vi "HV_mesura_Ileak.vi"(2 "VISA resource name":refnum<visa-resource-name>="GPIB1::25::INSTR", 3 "notifier Ileak":refnum<notifier>) -> ()   [LabVIEW 2015, in "VIPM2.lvlib"]
doc: "Executa segons notificacions les mesures de Ileak.\nEn acabar, grava CSV i les gràfiques en PNG dins de EQ folder path."
uses:
  VIPM2.lvlib
  dr_Keithley 24XX/Keithley 24XX.lvlib
panel:
  out "time":sgl
  out "barra":u8(slide) scale=0.0..5.0
  out "Waveform Graph":sgl[](graph)
  out "Chart":cluster{sgl, sgl}[](graph)
  out "Current":sgl format="%#_6p"
  out "Voltage":sgl
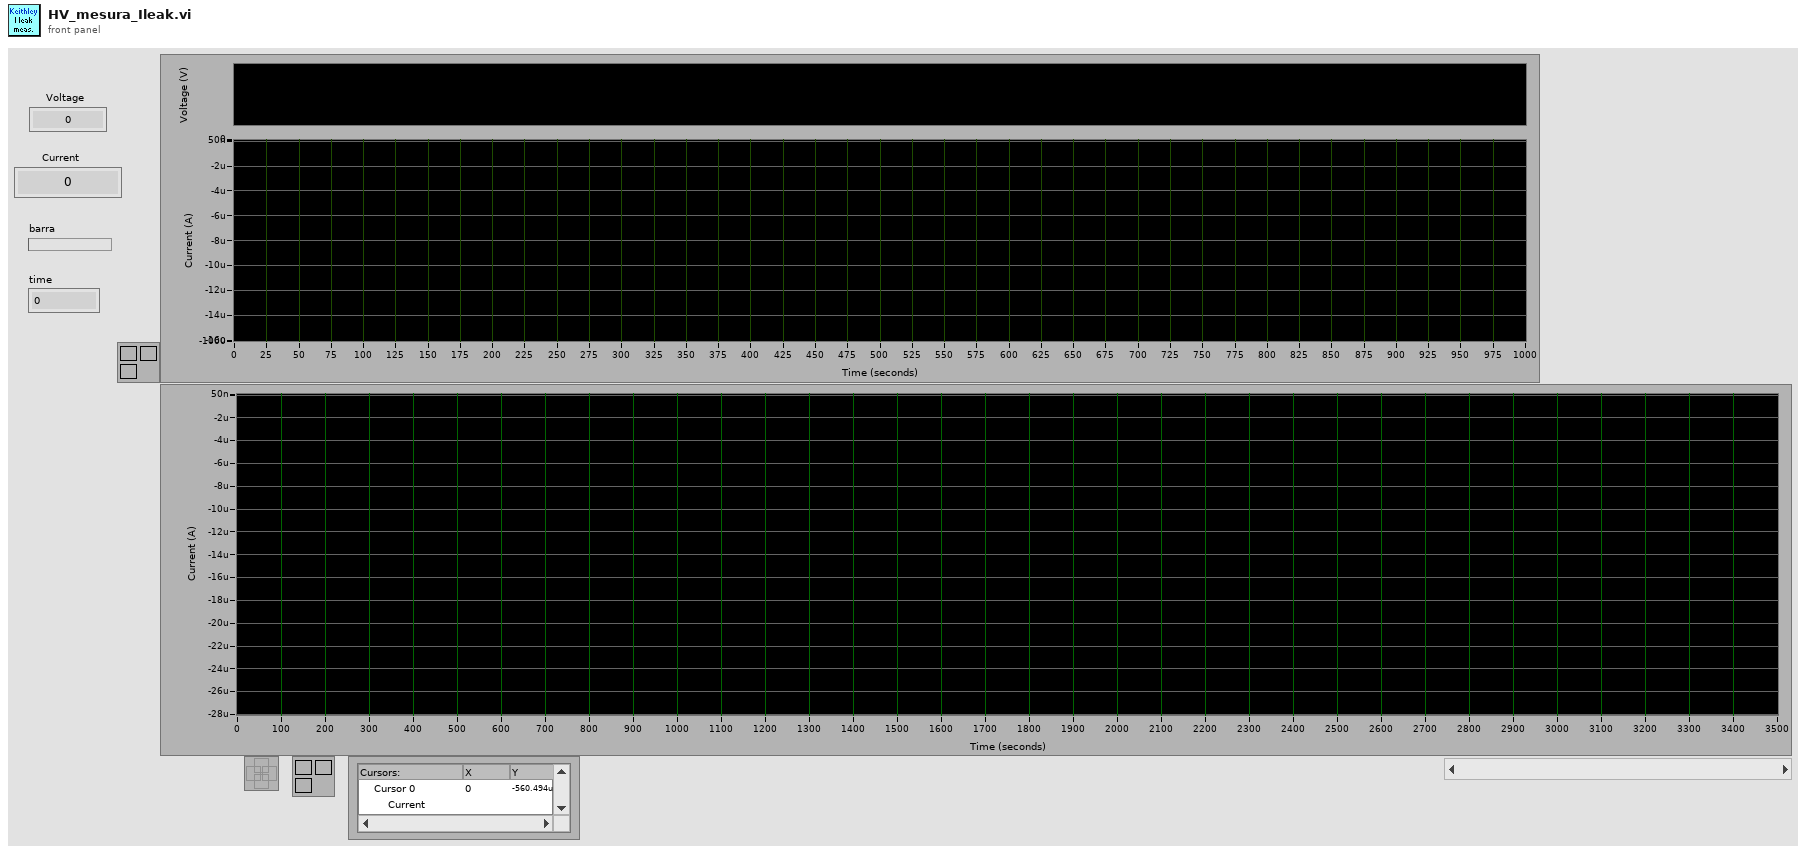
[diagram p1: front panel]
types:
  T1 = typedef "imagedata.ctl" = cluster{"image type":i32, "image depth":i32, "image":u8[], "mask":u8[], "colors":u32[], "Rectangle":cluster{"left":i16, "top":i16, "right":i16, "bottom":i16}}
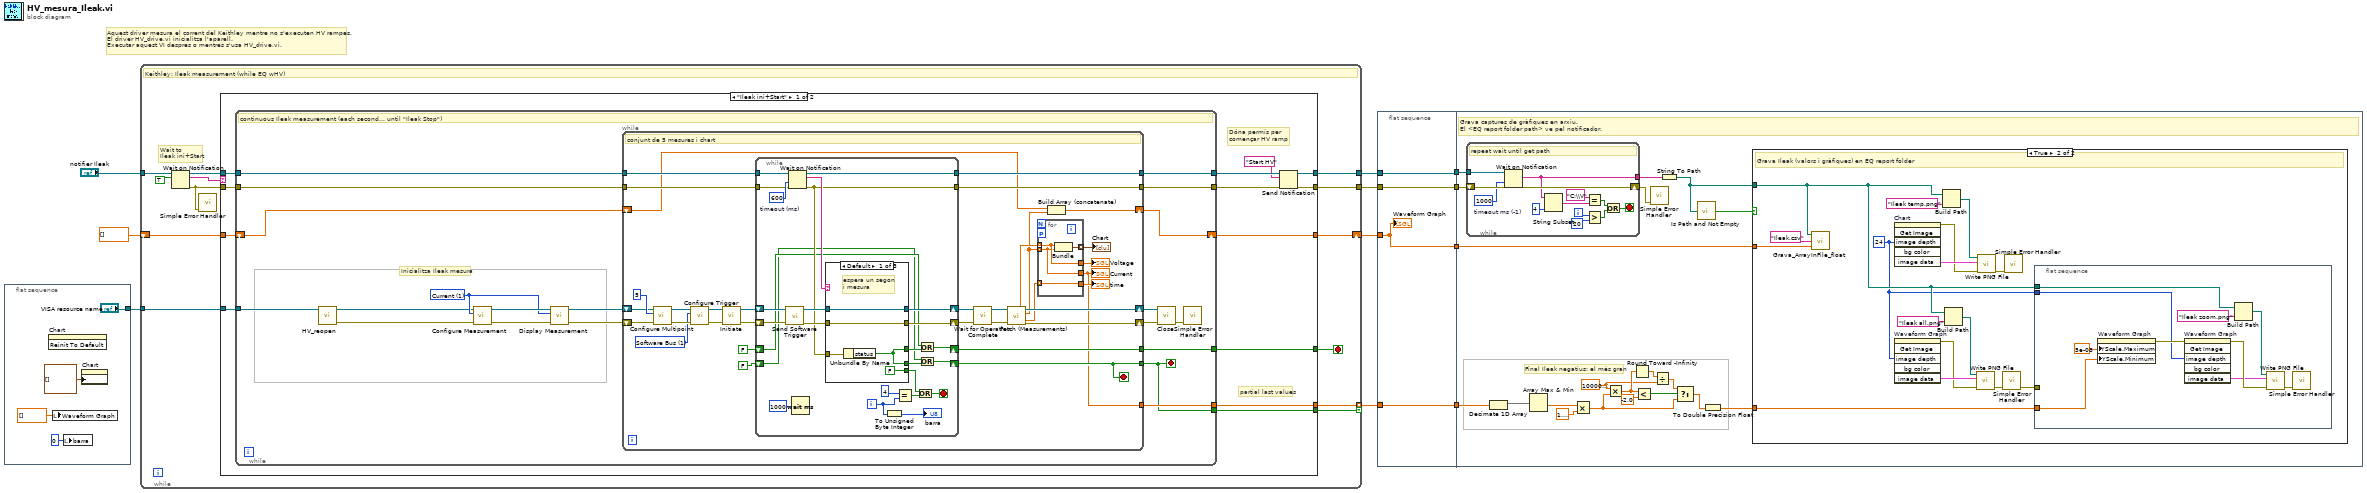
[diagram p0: block diagram]
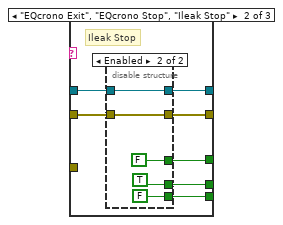
[diagram p3: hidden frame]
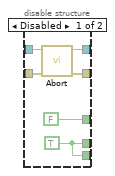
[diagram p4: hidden frame]
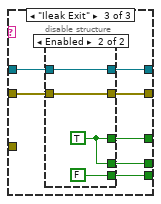
[diagram p5: hidden frame]
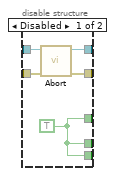
[diagram p6: hidden frame]
diagram:
  # "Aquest driver mesura el corrent del Keithley mentre no s'executen HV rampes.\nEl driver HV_drive.vi inicialitza l'aparell.\nExecutar aquest VI despres o mentres s'usa HV_drive.vi."
  n1 = flat-sequence {
    tunnel: ["VISA resource name"] -> w11
    frame #0 {
      n2 = invoke on="Chart" class="WFChart (strict)" method="Reinit To Default"() -> ()  [unwired: 3 in, 3 out]
      n3 = local write "Waveform Graph"(sgl[] [] ("Waveform Graph")) -> ()
      n4 = local write "barra"(u8 0 ("barra")) -> ()
      n5 = property on="Chart" class="WFChart (strict)"("History Data"=cluster{sgl, sgl}[] []) -> ()  [unwired: 2 in, 2 out]
    }
  }
  n6 = while {
    tunnel: w11 -> [w28]
    shift-right: [w27] -> w8
    shift-left: sgl[] [] -> [w26]
    tunnel: "notifier Ileak" -> [w25]
    tunnel: [w20] -> w7
    tunnel: [w19] -> w6
    tunnel: [w17] -> w2 mode=indexing if=w16
    stop <- w21 stop-if-true
    # "Wait to\nIleak ini+Start"
    # "Keithley: Ileak measurement (while EQ wHV)"
    n7 = Wait on Notification(notifier=w25, ignore previous (F)=TRUE) -> (notifier out=w22:refnum<notifier>, notification=w23:string, error out=w18:errorcluster)  [unwired: 2 in, 1 out]
    n8 = call <vilib>:"Simple Error Handler.vi"("error in (no error)"=w18) -> ()  [unwired: 4 in, 5 out]
    n9 = case shown="\"Ileak ini+Start\"" w23 {
      tunnel: w28 -> [w36 _]
      tunnel: [w41 w165] -> w27
      tunnel: w26 -> [w40 w165]
      tunnel: w22 -> [w39 w164]
      tunnel: w18 -> [w38 w163]
      tunnel: [w37 _] -> w21
      tunnel: [w34 w164] -> w20
      tunnel: [w32 w163] -> w19
      tunnel: [w30 _] -> w17
      tunnel: [w29 _] -> w16
      frame "Ileak ini+Start" {
        # "partial last values"
        # "Dóna permís per\ncomençar HV ramp"
        n10 = while {
          shift-right: [w57] -> w41
          shift-left: w40 -> [w55]
          tunnel: w39 -> [w61]
          tunnel: w38 -> [w60]
          tunnel: [w56] -> w37
          tunnel: [w59] -> w35
          tunnel: [w58] -> w33
          tunnel: w36 -> [w44]
          tunnel: [w46] -> w30
          tunnel: [w45] -> w29
          stop <- w45 stop-if-true
          w52 = u16 1 items=["Volts", "Current", "Resistance"] ("Function (0: Volts)")
          # "Inicialitza Ileak mesura"
          # "continuous Ileak measurement (each second... until \"Ileak Stop\")"
          n11 = call "HV_reopen.vi"("VISA resource name"=w44) -> ("error out"=w42:errorcluster, "VISA resource name out"=w43:refnum<visa-resource-name>)  [unwired: 9 in]
          n12 = call "Configure Measurement.vi"("error in (no error)"=w42, "Function (0: Volts)"=w52, "VISA resource name"=w43) -> ("error out"=w53:errorcluster, "VISA resource name out"=w54:refnum<visa-resource-name>)  [unwired: 7 in]
          n13 = call "Display Measurement.vi"("error in (no error)"=w53, "Displayed Measurement (0: Voltage)"=w52, "VISA resource name"=w54) -> ("error out"=w50:errorcluster, "VISA resource name out"=w51:refnum<visa-resource-name>)  [unwired: 7 in]
          n14 = while {
            tunnel: w61 -> [w76]
            tunnel: w60 -> [w75]
            tunnel: [w74] -> w59
            tunnel: [w73] -> w58
            tunnel: [w72] -> w56
            tunnel: [w71] -> w45
            shift-right: [w77] -> w57
            shift-left: w55 -> [w68]
            shift-right: [w94] -> w48
            shift-left: w51 -> [w67]
            shift-right: [w65] -> w47
            shift-left: w50 -> [w66]
            tunnel: [w64] -> w46
            stop <- w71 stop-if-true
            w91 = u16 1 items=["Immediate", "Software Bus", "Timer", "Manual", "Trigger Link", "Rising SOT Pulse", "Falling SOT Pulse", "Rising or Falling SOT Pulse"] ("Arming Source  (0: Immediate)")
            # "conjunt de 5 mesures i chart"
            n15 = call "Configure Multipoint.vi"("error in (no error)"=w66, "Number of Times to Arm (1)"=5 ("Trigger Count (1)"), "VISA resource name"=w67) -> ("error out"=w92:errorcluster, "VISA resource name out"=w93:refnum<visa-resource-name>)  [unwired: 7 in]
            n16 = call "Configure Trigger.vi"("error in (no error)"=w92, "Arming Source  (0: Immediate)"=w91, "VISA resource name"=w93) -> ("error out"=w89:errorcluster, "VISA resource name out"=w90:refnum<visa-resource-name>)  [unwired: 7 in]
            n17 = call "Initiate.vi"("error in (no error)"=w89, "VISA resource name"=w90) -> ("error out"=w87:errorcluster, "VISA resource name out"=w88:refnum<visa-resource-name>)  [unwired: 8 in]
            n18 = while {
              shift-right: [w104] -> w86
              shift-left: w88 -> [w118]
              shift-right: [w103] -> w85
              shift-left: w87 -> [w117]
              tunnel: w76 -> [w110]
              tunnel: w75 -> [w109]
              tunnel: [w107] -> w74
              tunnel: [w102] -> w73
              shift-right: [w98] -> w72
              shift-left: FALSE -> [w99]
              shift-right: [w95] -> w71
              shift-left: FALSE -> [w96]
              i -> [w113]
              stop <- w115 stop-if-true
              w111 = 600  # timeout (ms)
              n19 = call "Send Software Trigger.vi"("error in (no error)"=w117, "VISA resource name"=w118) -> ("error out"=w105:errorcluster, "VISA resource name out"=w106:refnum<visa-resource-name>)  [unwired: 8 in]
              n20 = Wait on Notification(notifier=w110, timeout in ms (-1)=w111, error in (no error)=w109) -> (notifier out=w107:refnum<notifier>, notification=w108:string, error out=w102:errorcluster)  [unwired: 1 in, 1 out]
              n21 = Wait (ms)(milliseconds to wait=u32 1000 ("millisecond multiple")) -> ()  [unwired: 1 out]
              n22 = case shown="Default" w108 {
                tunnel: w102 -> [w124 _ _]
                tunnel: [w121 w127 w145] -> w100
                tunnel: [w121 w126 w144] -> w97
                tunnel: w106 -> [w123 w131 w149]
                tunnel: w105 -> [w122 w130 w147]
                tunnel: [w123 w129 w148] -> w104
                tunnel: [w122 w128 w146] -> w103
                tunnel: [FALSE w125 w143] -> w101
                frame Default {
                  # "espera un segon\ni mesura"
                  n23 = Unbundle By Name(w124) -> ("status"=w121:bool)
                }
                frame "EQcrono Exit", "EQcrono Stop", "Ileak Stop" {
                  # "Ileak Stop"
                  n24 = disable-structure shown="Enabled" {
                    disable-tunnel: w131 -> [w137 w142]
                    disable-tunnel: w130 -> [w136 w141]
                    disable-tunnel: [w135 w142] -> w129
                    disable-tunnel: [w134 w141] -> w128
                    disable-tunnel: [FALSE FALSE] -> w127
                    disable-tunnel: [w132 TRUE] -> w126
                    disable-tunnel: [w132 FALSE] -> w125
                    frame Disabled {
                      w132 = TRUE
                      n25 = call "Abort.vi"("error in (no error)"=w136, "VISA resource name"=w137) -> ("error out"=w134:errorcluster, "VISA resource name out"=w135:refnum<visa-resource-name>)  [unwired: 8 in]
                    }
                    frame Enabled {
                    }
                  }
                }
                frame "Ileak Exit" {
                  n26 = disable-structure shown="Enabled" {
                    disable-tunnel: w149 -> [w154 w158]
                    disable-tunnel: [w153 w158] -> w148
                    disable-tunnel: w147 -> [w152 w157]
                    disable-tunnel: [w151 w157] -> w146
                    disable-tunnel: [w150 w156] -> w145
                    disable-tunnel: [w150 w156] -> w144
                    disable-tunnel: [w150 FALSE] -> w143
                    frame Disabled {
                      w150 = TRUE
                      n27 = call "Abort.vi"("error in (no error)"=w152, "VISA resource name"=w154) -> ("error out"=w151:errorcluster, "VISA resource name out"=w153:refnum<visa-resource-name>)  [unwired: 8 in]
                    }
                    frame Enabled {
                      w156 = TRUE
                    }
                  }
                }
              }
              n28 = To Unsigned Byte Integer(number=w113) -> (unsigned 8bit integer=→"barra":u8)
              n29 = Equal?(x=4 ("y"), y=w113) -> (x = y?=w116:bool)
              n30 = Or(x=w101, y=w116) -> (x .or. y?=w115:bool)
              n31 = Or(x=w96, y=w97) -> (x .or. y?=w95:bool)
              n32 = Or(x=w99, y=w100) -> (x .or. y?=w98:bool)
            }
            n33 = call "Wait for Operation Complete.vi"("error in (no error)"=w85, "VISA resource name"=w86) -> ("error out"=w83:errorcluster, "VISA resource name out"=w84:refnum<visa-resource-name>)  [unwired: 8 in]
            n34 = call "Fetch (Measurements).vi"("VISA resource name"=w84, "error in (no error)"=w83) -> ("Voltage"=w81:sgl[], "VISA resource name out"=w94:refnum<visa-resource-name>, "Current"=w78:sgl[], "Timestamp"=w70:sgl[], "error out"=w65:errorcluster)  [unwired: 7 in, 2 out]
            n35 = for {
              tunnel: w81 -> [w161] mode=indexing
              tunnel: w78 -> [w160] mode=indexing
              tunnel: [w162] -> w80 mode=indexing
              tunnel: [w161] -> w79
              tunnel: [w160] -> w64
              tunnel: w70 -> [w159] mode=indexing
              tunnel: [w159] -> w69
              workers-P: _ -> [_]
              n36 = Bundle(w161, w160) -> (w162:cluster{sgl, sgl})  [unwired: 1 in]
            }
            "Chart" <- w80
            "Voltage" <- w79
            "Current" <- w64
            "time" <- w69
            n37 = Build Array (concatenate) "Build Array"(w68, w78) -> (w77:sgl[])
          }
          n38 = call "Close.vi"("error in (no error)"=w47, "VISA resource name"=w48) -> ("error out"=w49:errorcluster)  [unwired: 9 in]
          n39 = call <vilib>:"Simple Error Handler.vi"("error in (no error)"=w49) -> ()  [unwired: 4 in, 5 out]
        }
        n40 = Send Notification(notification="Start HV", notifier=w35, error in (no error)=w33) -> (notifier out=w34:refnum<notifier>, error out=w32:errorcluster)
      }
      frame Default {
      }
    }
  }
  n41 = flat-sequence {
    tunnel: w8 -> [w167]
    tunnel: w7 -> [w169]
    tunnel: w6 -> [w168]
    tunnel: [w169] -> w5
    tunnel: [w168] -> w4
    tunnel: [w167] -> w3
    tunnel: w2 -> [w166]
    tunnel: [w166] -> w1
    tunnel: w5 -> [w189]
    tunnel: w4 -> [w188]
    tunnel: w3 -> [w184]
    tunnel: w1 -> [w182]
    frame #0 {
      "Waveform Graph" <- w167
    }
    frame #1 {
      w173 = sgl 1000000.0 ("x")
      # "Final Ileak negatius: el més gran"
      # "Grava captures de gràfiques en arxiu.\nEl <EQ report folder path> ve pel notificador."
      n42 = while {
        tunnel: w189 -> [w202]
        tunnel: [w198] -> w186
        shift-right: [w199] -> w187
        shift-left: w188 -> [w201]
        i -> [w194]
        stop <- w190 stop-if-true
        w200 = 1000  # timeout ms (-1)
        # "repeat wait until get path"
        n43 = Wait on Notification(notifier=w202, timeout in ms (-1)=w200, error in (no error)=w201) -> (notification=w198:string, error out=w199:errorcluster)  [unwired: 1 in, 2 out]
        n44 = String Subset(string=w198, length (rest)=4 ("length (rest)")) -> (substring=w196:string)  [unwired: 1 in]
        n45 = Equal?(x="C:\\V", y=w196) -> (x = y?=w191:bool)
        n46 = Greater?(x=w194, y=20) -> (0:w192:bool)
        n47 = Or(x=w191, y=w192) -> (x .or. y?=w190:bool)
      }
      n48 = Decimate 1D Array "Decimate 1D Array"(w182) -> (w181:sgl[])  [unwired: 1 out]
      n49 = Array Max & Min(array=w181) -> (min value=w180:sgl)  [unwired: 3 out]
      n50 = Multiply(x=w180, y=sgl 1.2) -> (x*y=w171:sgl)
      n51 = Multiply(x=w173, y=w171) -> (x*y=w175:sgl)
      n52 = Round Toward -Infinity(1:w175) -> (0:w174:sgl)
      n53 = Less?(x=w175, y=sgl -2.0) -> (x < y?=w177:bool)
      n54 = call <vilib>:"Simple Error Handler.vi"("error in (no error)"=w187) -> ()  [unwired: 4 in, 5 out]
      n55 = Divide(x=w174, y=w173) -> (x/y=w172:sgl)
      n56 = String To Path(string=w186) -> (path=w183:path)
      n57 = Select(t=w172, s=w177, f=w171) -> (s? t:f=w170:sgl)
      n58 = call <vilib>:"Is Path and Not Empty.vi"("path"=w183) -> ("Is Path and Not Empty?"=w185:bool)  [unwired: 4 in]
      n59 = To Double Precision Float(number=w170) -> (double precision float=w178:dbl)
      n60 = case shown="True" w185 {
        tunnel: w184 -> [_ w218]
        tunnel: w183 -> [_ w205]
        tunnel: w178 -> [_ w203]
        frame False {
          # "no és path"
        }
        frame True {
          w204 = 24 ("Image Depth")
          # "Grava Ileak (valors i gràfiques) en EQ report folder"
          n61 = call "Grava_ArrayInFile_float.vi"("Array to save"=w218, "file name"="Ileak.csv", "folder path"=w205) -> ()  [unwired: 2 in]
          n62 = invoke on="Chart" class="WFChart (strict)" method="Get Image"("image depth"=w204) -> (error out=w215:errorcluster, "image data"=w216:T1)  [unwired: 5 in, 4 out]
          n63 = invoke on="Waveform Graph" class="WFGraph (strict)" method="Get Image"("image depth"=w204) -> (error out=w209:errorcluster, "image data"=w210:T1)  [unwired: 5 in, 4 out]
          n64 = Build Path(base path=w205, name or relative path="Ileak temp.png") -> (appended path=w213:path)
          n65 = Build Path(base path=w205, name or relative path="Ileak all.png") -> (appended path=w207:path)
          n66 = call <vilib>:"Write PNG File.vi"("error in (no error)"=w209, "image data"=w210, "path to PNG file"=w207) -> ("error out"=w211:errorcluster)  [unwired: 7 in, 1 out]
          n67 = call <vilib>:"Write PNG File.vi"("error in (no error)"=w215, "image data"=w216, "path to PNG file"=w213) -> ("error out"=w212:errorcluster)  [unwired: 7 in, 1 out]
          n68 = call <vilib>:"Simple Error Handler.vi"("error in (no error)"=w211) -> ("error out"=w206:errorcluster)  [unwired: 4 in, 4 out]
          n69 = call <vilib>:"Simple Error Handler.vi"("error in (no error)"=w212) -> ()  [unwired: 4 in, 5 out]
          n70 = flat-sequence {
            tunnel: w206 -> [_]
            tunnel: w205 -> [w221]
            tunnel: w204 -> [w220]
            tunnel: w203 -> [w219]
            frame #0 {
              n71 = property on="Waveform Graph" class="WFGraph (strict)"("YScale.Maximum"=5e-08 ("Y Scale.Range:Maximum"), "YScale.Minimum"=w219) -> (error out=w222:errorcluster)  [unwired: 2 in, 1 out]
              n72 = invoke on="Waveform Graph" class="WFGraph (strict)" method="Get Image"(error in=w222, "image depth"=w220) -> (error out=w225:errorcluster, "image data"=w224:T1)  [unwired: 4 in, 4 out]
              n73 = Build Path(base path=w221, name or relative path="Ileak zoom.png") -> (appended path=w227:path)
              n74 = call <vilib>:"Write PNG File.vi"("error in (no error)"=w225, "image data"=w224, "path to PNG file"=w227) -> ("error out"=w223:errorcluster)  [unwired: 7 in, 1 out]
              n75 = call <vilib>:"Simple Error Handler.vi"("error in (no error)"=w223) -> ()  [unwired: 4 in, 5 out]
            }
          }
        }
      }
    }
  }
